vi "_Operate.vi"(7 "DB Ref":T1, 8 "error in (no error)":errorcluster, 9 "parameter":string, 10 "Operation":string, 11 "Ctrl":string) -> (0 "error out":errorcluster)   [LabVIEW 2017, in "TagDB RefManager.lvlib"]
uses:
  TagDB RefManager.lvlib
  <userlib>/_NEVSTOP/TagDB/Typedef/TagDB.ctl
  _Opers/tagdb-RefMgr Operations.lvlib
  <userlib>/_NEVSTOP/TagDB/TagDB.lvlib
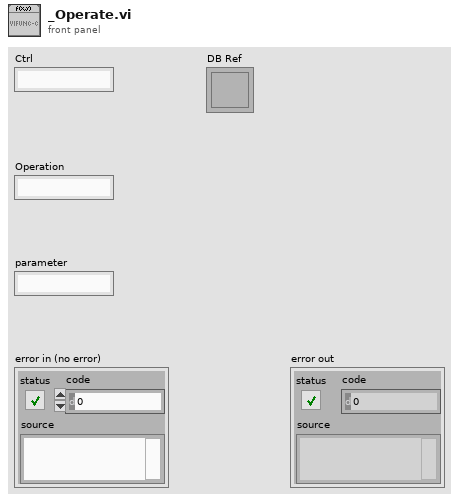
[diagram p1: front panel]
types:
  T1 = typedef "TagDB.lvlib/TagDB.ctl" = refnum<k1>
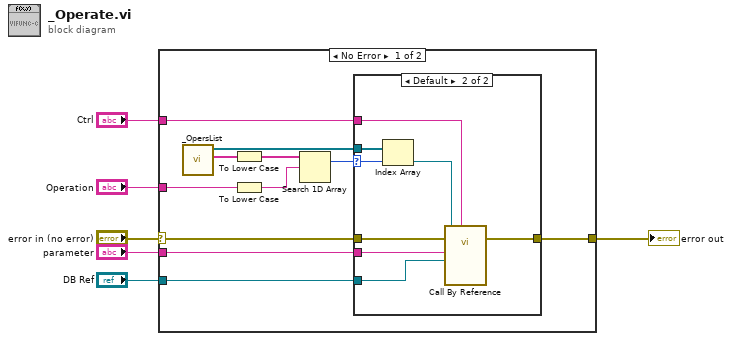
[diagram p0: block diagram]
diagram:
  n1 = case shown="No Error" "error in (no error)" {
    selector: "error in (no error)" -> [w15 w27]
    tunnel: "Operation" -> [w17 _]
    tunnel: [w14 w27] -> w4
    tunnel: "parameter" -> [w13 _]
    tunnel: "Ctrl" -> [w12 _]
    tunnel: "DB Ref" -> [w11 _]
    frame No Error {
      n2 = call "_OpersList.vi"() -> ("built-in VIFuncs"=w9:string[], "Array"=w10:refnum<vi>[])  [unwired: 9 in, 1 out]
      n3 = To Lower Case(string=w9) -> (all lower case string=w8:string[])
      n4 = To Lower Case(string=w17) -> (all lower case string=w7:string)
      n5 = Search 1D Array(1D array=w8, element=w7) -> (index of element=w16:i32)  [unwired: 1 in]
      n6 = case shown="Default" w16 {
        selector: w16 -> [_ w25]
        tunnel: w10 -> [_ w26]
        tunnel: w15 -> [w18 w24]
        tunnel: [w18 w23] -> w14
        tunnel: w13 -> [_ w21]
        tunnel: w12 -> [_ w20]
        tunnel: w11 -> [_ w19]
        frame -1 {
        }
        frame Default {
          n7 = Index Array(array=w26, index=w25) -> (element=w22:refnum<vi>)
          n8 = call-by-ref "?"(reference=w22, error in=w24, "Ctrl"=w20, "TagDB"=w19, "String"=w21) -> (error out=w23:errorcluster)  [unwired: 8 in, 2 out]
        }
      }
    }
    frame Error {
    }
  }
  "error out" <- w4
